vi "Timer_Global.vi"(7 "Timer Action (Get) (In)":T1=enum."Get", 8 "Error In":errorcluster, 11 "Timer ID (0) (In)":i32 min=0) -> (0 "Error Out":errorcluster, 2 "Time Difference":dbl, 3 "Timer ID (Out)":i32 min=0)   [LabVIEW 2014]
uses:
  Timer_Global_Action_Control.ctl
panel:
  out "Caller List (Out)":string[][](array[string])
  out "Timestamps (Out)":timestamp[][](array[timestamp])
  out "ID List (Out)":i32[][](array[numeric])
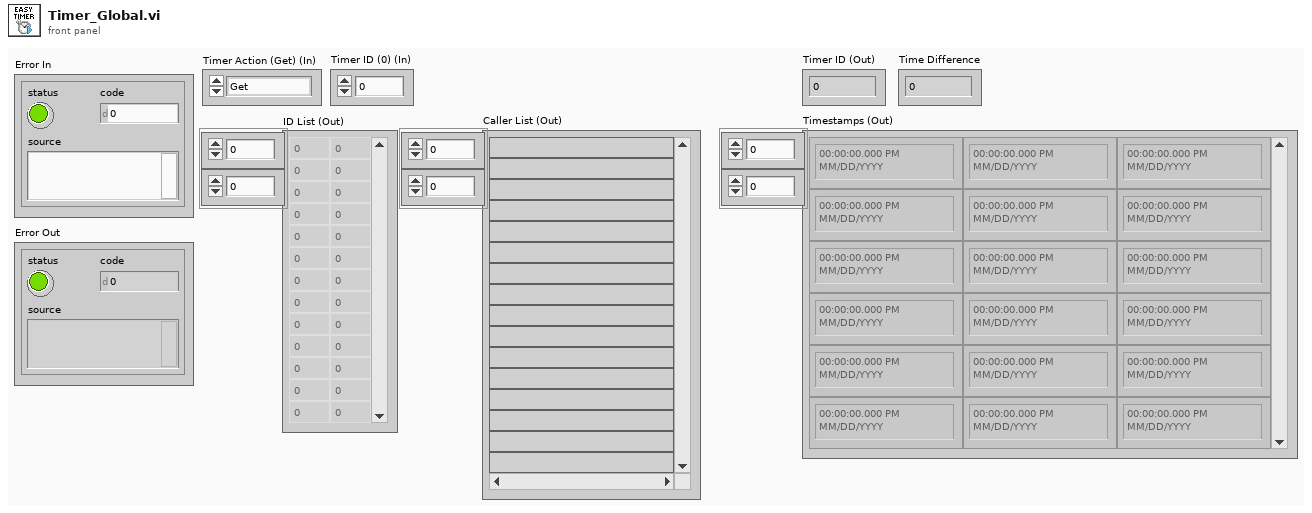
[diagram p1: front panel]
types:
  T1 = typedef "Timer_Global_Action_Control.ctl" = enum16{"Init", "Set", "Get", "Update", "Clear"}
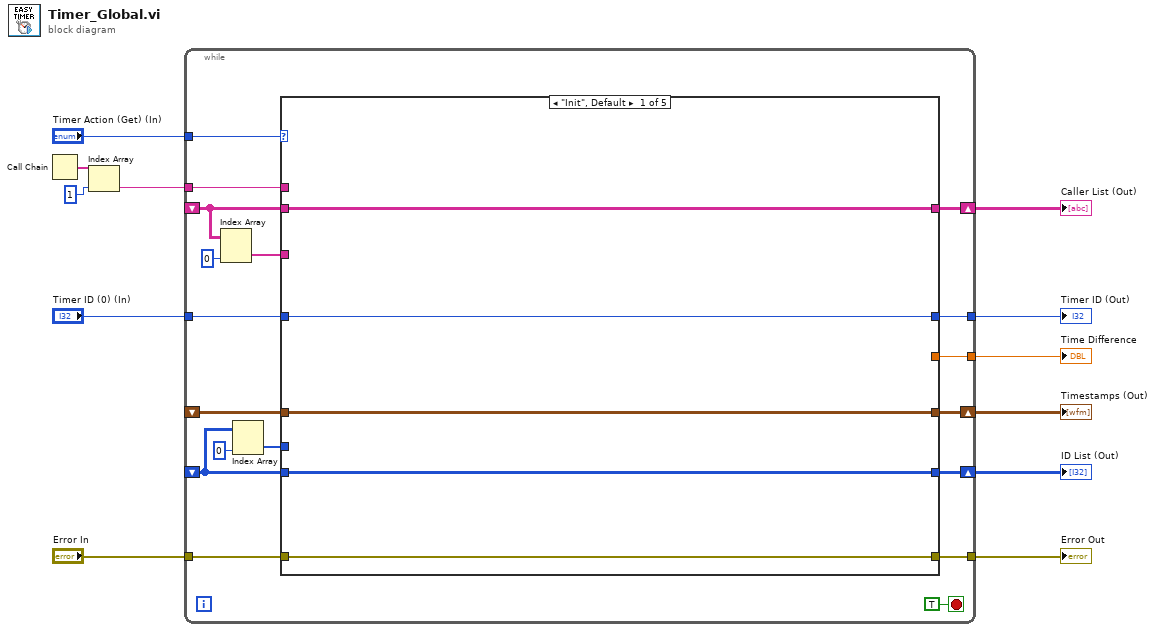
[diagram p0: block diagram]
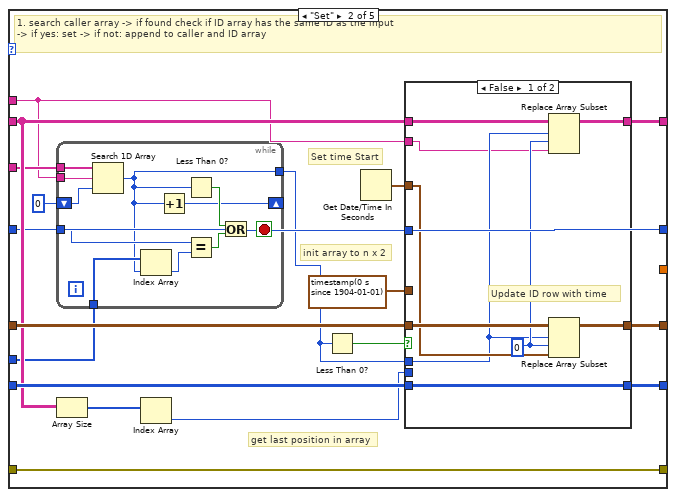
[diagram p2: hidden frame]
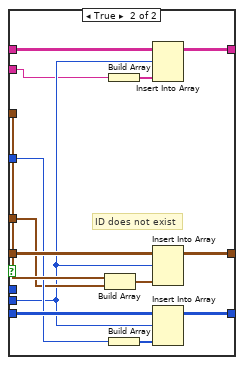
[diagram p3: hidden frame]
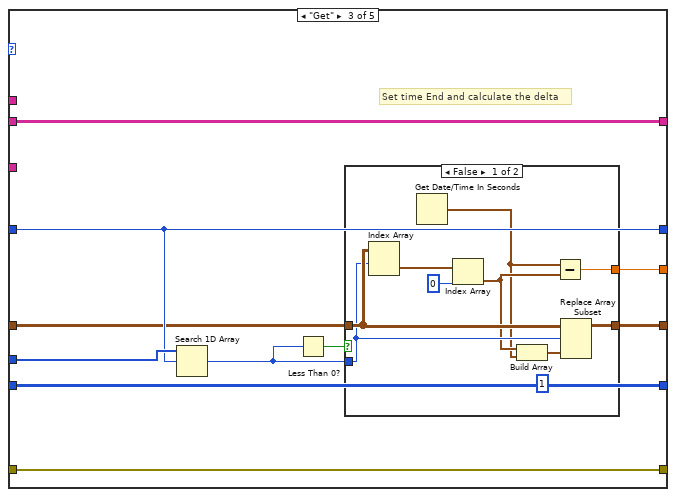
[diagram p4: hidden frame]
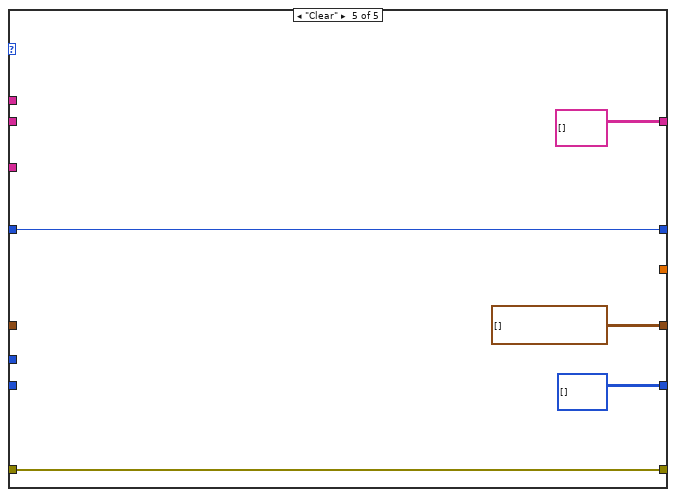
[diagram p7: hidden frame]
diagram:
  n1 = Call Chain() -> (call chain=w3:string[])
  n2 = Index Array(array=w3, index=1) -> (element=w1:string)
  n3 = while {
    tunnel: "Timer Action (Get) (In)" -> [w29]
    tunnel: [w26] -> w10
    tunnel: "Timer ID (0) (In)" -> [w25]
    tunnel: [w22] -> w7
    shift-right: [w27] -> w11
    shift-left: _ -> [w17]
    shift-right: [w28] -> w8
    shift-left: _ -> [w24]
    tunnel: [w20] -> w6
    tunnel: "Error In" -> [w19]
    shift-right: [w18] -> w4
    shift-left: _ -> [w15]
    tunnel: w1 -> [w13]
    stop <- TRUE stop-if-true
    n4 = Index Array(array=w15, index (col)=0 ("disabled index (col)")) -> (element=w14:string[])  [unwired: 1 in]
    n5 = Index Array(array=w17, index (col)=0 ("disabled index (col)")) -> (element=w23:i32[])  [unwired: 1 in]
    n6 = case shown="\"Init\", Default" w29 {
      tunnel: [w35 w53 w93 w112 timestamp[][] [] ("Timestamps Default")] -> w28
      tunnel: w24 -> [w35 w52 w94 w112 _]
      tunnel: [w34 w49 w97 w111 i32[][] [] ("ID List")] -> w27
      tunnel: w17 -> [w34 w48 w97 w111 _]
      tunnel: [w33 w38 w95 w110 w117] -> w26
      tunnel: w25 -> [w33 w38 w95 w110 w117]
      tunnel: w23 -> [_ w39 w96 _ _]
      tunnel: [_ _ w92 _ _] -> w22
      tunnel: [w32 w44 w89 w109 w114] -> w20
      tunnel: w19 -> [w32 w44 w89 w109 w114]
      tunnel: [w31 w43 w88 w108 string[][] [] ("Caller List (Out)")] -> w18
      tunnel: w15 -> [w31 w42 w88 w108 _]
      tunnel: w14 -> [_ w41 _ _ _]
      tunnel: w13 -> [_ w40 _ _ _]
      frame "Init", Default {
      }
      frame "Set" {
        # "get last position in array"
        # "init array to n x 2"
        # "Set time Start"
        # "1. search caller array -> if found check if ID array has the same ID as the input\n-> if yes: set -> if not: append to caller and ID array"
        n7 = while {
          tunnel: w41 -> [w62]
          tunnel: w40 -> [w55]
          tunnel: w39 -> [w64]
          tunnel: w38 -> [w63]
          shift-right: [w56] -> _
          shift-left: 0 ("index (col)") -> [w61]
          tunnel: [w54] -> w36
          stop <- w58 stop-if-true
          n8 = Search 1D Array(1D array=w62, element=w55, start index (0)=w61) -> (index of element=w54:i32)
          n9 = Index Array(array=w64, index=w54) -> (element=w60:i32)
          n10 = Increment(x=w54) -> (x+1=w56:i32)
          n11 = Less Than 0?(x=w54) -> (x < 0?=w57:bool)
          n12 = Equal?(x=w63, y=w60) -> (x = y?=w59:bool)
          n13 = Or(x=w57, y=w59) -> (x .or. y?=w58:bool)
        }
        n14 = Array Size(array=w42) -> (size(s)=w47:i32[])
        n15 = Index Array(array=w47) -> (element=w46:i32)  [unwired: 1 in]
        n16 = Less Than 0?(x=w36) -> (x < 0?=w50:bool)
        n17 = Get Date/Time In Seconds() -> (seconds since 1Jan1904=w51:timestamp)
        n18 = case shown="False" w50 {
          tunnel: [w73 w86] -> w53
          tunnel: w52 -> [w72 w87]
          tunnel: w51 -> [w71 w84]
          tunnel: w36 -> [w66 _]
          tunnel: w48 -> [w70 w83]
          tunnel: [w70 w82] -> w49
          tunnel: w46 -> [_ w76]
          tunnel: w38 -> [_ w80]
          tunnel: timestamp(0 s since 1904-01-01) ("element") -> [_ w79]
          tunnel: w42 -> [w69 w77]
          tunnel: [w68 w78] -> w43
          tunnel: w40 -> [w65 w75]
          frame False {
            w67 = 0 ("index (col)")
            # "Update ID row with time"
            n19 = Replace Array Subset(array=w69, new element=w65, index (row)=w66, index (col)=w67) -> (w68:string[][])
            n20 = Replace Array Subset(array=w72, new element=w71, index (row)=w66, index (col)=w67) -> (w73:timestamp[][])
          }
          frame True {
            # "ID does not exist"
            n21 = Build Array(w84, w79) -> (w85:timestamp[])
            n22 = Build Array(w75) -> (w74:string[])
            n23 = Build Array(w80) -> (w81:i32[])
            n24 = Insert Into Array(array=w77, index (row)=w76, new element=w74) -> (w78:string[][])  [unwired: 1 in]
            n25 = Insert Into Array(array=w87, index (row)=w76, new element=w85) -> (w86:timestamp[][])  [unwired: 1 in]
            n26 = Insert Into Array(array=w83, index (row)=w76, new element=w81) -> (w82:i32[][])  [unwired: 1 in]
          }
        }
      }
      frame "Get" {
        # "Set time End and calculate the delta"
        n27 = Search 1D Array(1D array=w96, element=w95) -> (index of element=w91:i32)  [unwired: 1 in]
        n28 = Less Than 0?(x=w91) -> (x < 0?=w90:bool)
        n29 = case shown="False" w90 {
          tunnel: w94 -> [w104 w107]
          tunnel: [w103 w107] -> w93
          tunnel: w91 -> [w102 _]
          tunnel: [w101 _] -> w92
          frame False {
            (unwired) 1 ("disabled index (col)")
            n30 = Index Array(array=w104, index (row)=w102) -> (element=w106:timestamp[])  [unwired: 1 in]
            n31 = Get Date/Time In Seconds() -> (seconds since 1Jan1904=w98:timestamp)
            n32 = Index Array(array=w106, index=0 ("disabled index (col)")) -> (element=w99:timestamp)
            n33 = Build Array(w99, w98) -> (w100:timestamp[])
            n34 = Subtract(x=w98, y=w99) -> (x-y=w101:dbl)
            n35 = Replace Array Subset(array=w104, new element=w100, index (row)=w102) -> (w103:timestamp[][])  [unwired: 1 in]
          }
          frame True {
          }
        }
      }
      frame "Update" {
      }
      frame "Clear" {
      }
    }
  }
  "ID List (Out)" <- w11
  "Error Out" <- w6
  "Time Difference" <- w7
  "Timer ID (Out)" <- w10
  "Timestamps (Out)" <- w8
  "Caller List (Out)" <- w4
